vi "Get CurrentElement.vi"(8 "error in (no error)":errorcluster, 11 "CircularBuffer":refnum<class "CircularBuffer.lvclass">) -> (0 "error out":errorcluster, 2 "Element":variant, 3 "CircularBuffer out":refnum<class "CircularBuffer.lvclass">)   [LabVIEW 2016, in "CircularBuffer.lvclass"]
doc: "---------------------------------------------------------------\nJKI State Machine Objects™\nhttp://jki.net/state-machine-objects/\nCopyright (C) 2005-2015, JKI <info@jki.net>\nALL RIGHTS RESERVEDJKI State Machine Objects (SMO) 1.0.0.4\nJKI - JKI\nCopyright (c) 2015, JKI"
uses:
  CircularBuffer.lvclass
  types/type/type.lvclass
panel:
  # "For instructions on how to use the JKI State Machine Objects, examples and video tutorials, visit:\nhttp://jki.net/state-machine-objects/\n\nJKI State Machine Objects™\nhttp://jki.net/state-machine-objects/\nCopyright (C) 2005-2015, JKI <info@jki.net>\nALL RIGHTS RESERVED"
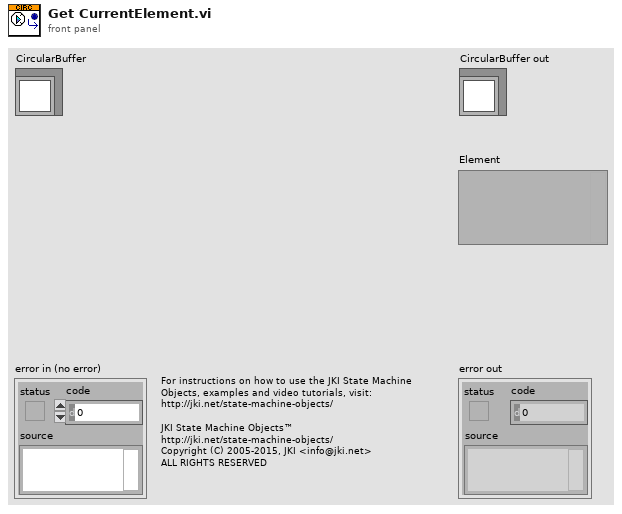
[diagram p1: front panel]
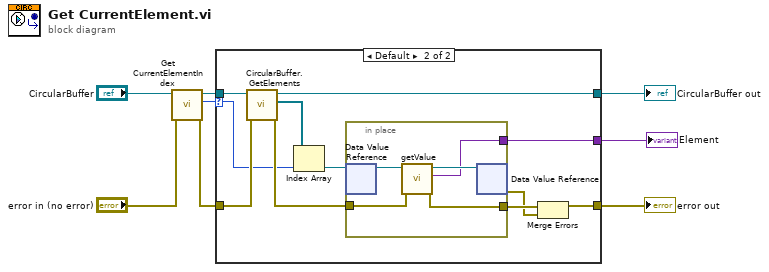
[diagram p0: block diagram]
diagram:
  n1 = call "Get CurrentElementIndex.vi"("error in (no error)"="error in (no error)", "CircularBuffer"="CircularBuffer") -> ("error out"=w2:errorcluster, "Current Element index"=w1:i32, "CircularBuffer out"=w4:refnum<class "CircularBuffer.lvclass">)  [unwired: 7 in]
  n2 = case shown="Default" w1 {
    selector: w1 -> [_ w11]
    tunnel: [w10 w21] -> w8
    tunnel: [w9 w20] -> w7
    tunnel: [_ w19] -> w6
    tunnel: w4 -> [w10 w13]
    tunnel: w2 -> [w9 w12]
    frame -1 {
    }
    frame Default {
      n3 = call "CircularBuffer.GetElements.vi"("error in (no error)"=w12, "CircularBuffer in"=w13) -> ("error out"=w16:errorcluster, "Elements"=w18:refnum<data-value>[], "CircularBuffer out"=w21:refnum<class "CircularBuffer.lvclass">)  [unwired: 7 in]
      n4 = Index Array(array=w18, index=w11) -> (element=w17:refnum<data-value>)
      n5 = in-place {
        in-place-border: [w24] -> w19
        in-place-border: w16 -> [w23]
        in-place-border: [w22] -> w15
        n6 = in-place-dvr #1(w17) -> (w26:refnum<class "type.lvclass">)  [unwired: 1 out]
        n7 = call-dynamic "getValue.vi"("error in (no error)"=w23, "type in"=w26) -> ("error out"=w22:errorcluster, "value"=w24:variant, "type out"=w25:refnum<class "type.lvclass">)  [unwired: 7 in]
        n8 = in-place-dvr #1(w25) -> (w14:errorcluster)  [unwired: 1 out]
      }
      n9 = Merge Errors(w15, w14) -> (w20:errorcluster)
    }
  }
  "error out" <- w7
  "CircularBuffer out" <- w8
  "Element" <- w6
